vi "Handle Last Ack Core.vi"(4 "error in (no error)":errorcluster, 6 "Last Ack":refnum<class "Last Ack.lvclass">, 7 "Caller in":refnum<class "Caller.lvclass">) -> (0 "error out":errorcluster, 3 "Caller out":refnum<class "Caller.lvclass">)   [LabVIEW 2020, in "Caller.lvlib" / "Caller.lvclass"]
doc: "(<B>Filename</B>: Actor Framework.lvlib:Actor.lvclass:Handle Last Ack Core.vi)\n\nDefines how the caller actor responds to the Last Ack message from a nested actor. The Last Ack message is the final message a nested actor sends to its caller before it shuts down. The message contains information about the final state of the nested actor.\n\nBy default, this method does nothing except return any error the nested actor sent. A descendant class may override this method to define behavior."
uses:
  Caller.lvclass
  <vilib>/ActorFramework/LastAck/Last Ack.lvclass
  Nested/Nested.lvclass
  <vilib>/ActorFramework/LastAck/Last Ack.lvclass/Last Ack.ctl
  Nested/Nested.lvclass/Nested.ctl
  Caller.lvclass/Caller.ctl
  <vilib>/ActorFramework/Message Enqueuer/Message Enqueuer.lvclass/Message Enqueuer.ctl
  399a52ab-de9c-4f47-9720-846dc4beb769.vi
  Nested/Read Numeric.vi
  399a52ab-de9c-4f47-9720-846dc4beb769.vi/d4db2432-cc9c-482c-8957-dac855435ef6.vi
  399a52ab-de9c-4f47-9720-846dc4beb769.vi/86fbf154-bd7b-49a2-8ab2-a837b2a95f24.vi
  399a52ab-de9c-4f47-9720-846dc4beb769.vi/3b95b01e-1ec2-4565-bcd9-7606a5281010.vi
  399a52ab-de9c-4f47-9720-846dc4beb769.vi/96a08935-737a-44b2-979c-a81d56408f7e.vi
  <vilib>/ActorFramework/Message Enqueuer/Enqueue.vi
  399a52ab-de9c-4f47-9720-846dc4beb769.vi/d4db2432-cc9c-482c-8957-dac855435ef6.vi/6eaecd13-6e48-4772-a921-b51ebdf84d88.vi
  399a52ab-de9c-4f47-9720-846dc4beb769.vi/d4db2432-cc9c-482c-8957-dac855435ef6.vi/d2d5f2b7-06f4-47f6-971c-049c3fdbb653.vi
  399a52ab-de9c-4f47-9720-846dc4beb769.vi/3b95b01e-1ec2-4565-bcd9-7606a5281010.vi/6eaecd13-6e48-4772-a921-b51ebdf84d88.vi
  399a52ab-de9c-4f47-9720-846dc4beb769.vi/3b95b01e-1ec2-4565-bcd9-7606a5281010.vi/d2d5f2b7-06f4-47f6-971c-049c3fdbb653.vi
  399a52ab-de9c-4f47-9720-846dc4beb769.vi/96a08935-737a-44b2-979c-a81d56408f7e.vi/6eaecd13-6e48-4772-a921-b51ebdf84d88.vi
  399a52ab-de9c-4f47-9720-846dc4beb769.vi/96a08935-737a-44b2-979c-a81d56408f7e.vi/d2d5f2b7-06f4-47f6-971c-049c3fdbb653.vi
  Caller Messages/UpdateCPTNested Msg/UpdateCPTNested Msg.lvclass
  C:/Program Files/National Instruments/LabVIEW 2020/vi.lib/ActorFramework/Message/Message.lvclass
  <vilib>/ActorFramework/Message Priority Queue/Priority Enqueue.vi
  <vilib>/ActorFramework/Actor/Actor.lvclass
  <vilib>/Comparison/Less/Less Functor/Less Functor.lvclass
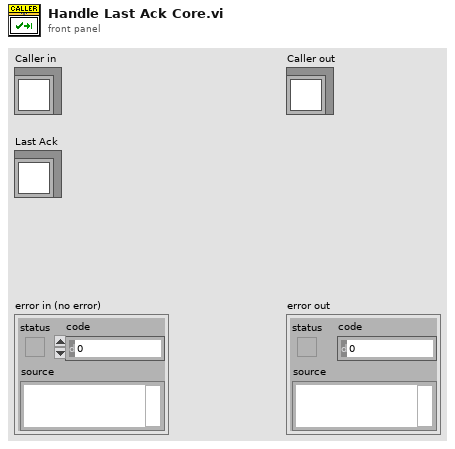
[diagram p1: front panel]
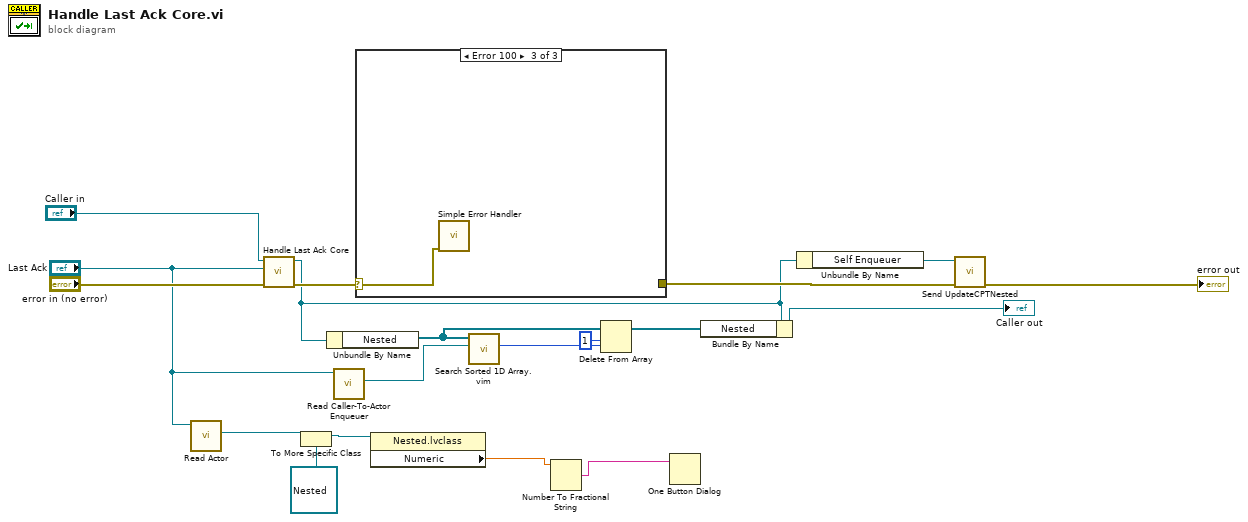
[diagram p0: block diagram]
diagram:
  n1 = call <vilib>:"Read Actor.vi"("Last Ack"="Last Ack") -> ("Actor"=w3:refnum<class "Actor.lvclass">)  [unwired: 10 in]
  n2 = call-parent "Handle Last Ack Core.vi"("error in (no error)"="error in (no error)", "Last Ack"="Last Ack", "Actor in"="Caller in") -> ("error out"=w9:errorcluster, "Actor out"=w7:refnum<class "Caller.lvclass">)  [unwired: 3 in]
  n3 = To More Specific Class(target class=refnum<class "Nested.lvclass"> refnum ("Nested.lvlib:Nested.lvclass"), reference=w3) -> (specific class reference=w4:refnum<class "Nested.lvclass">)  [unwired: 1 in, 1 out]
  n4 = Unbundle By Name(w7) -> ("Nested"=w14:refnum<class "Message Enqueuer.lvclass">[])
  n5 = call <vilib>:"Read Caller-To-Actor Enqueuer.vi"("Last Ack"="Last Ack") -> ("Caller-to-Actor Enqueuer"=w15:refnum<class "Message Enqueuer.lvclass">)  [unwired: 10 in]
  n6 = case shown="Error 100" w9 {
    selector: w9 -> [w20 w21 w22]
    tunnel: [w20 w21 _] -> w8
    frame No Error {
    }
    frame Default {
    }
    frame Error {
      n7 = call <vilib>:"Simple Error Handler.vi"("error in (no error)"=w22) -> ()  [unwired: 4 in, 5 out]
    }
  }
  n8 = property class="Nested.lvclass"(reference=w4) -> ("Numeric"=w2:dbl)  [unwired: 1 in, 2 out]
  n9 = call "Search Sorted 1D Array.vim"("element"=w15, "sorted 1D array"=w14) -> ("nearest index"=w13:i32)  [unwired: 8 in, 1 out]
  n10 = Number To Fractional String(number=w2) -> (F-format string=w1:string)  [unwired: 3 in]
  n11 = Delete From Array(array=w14, length=1, index=w13) -> (array with subset deleted=w10:refnum<class "Message Enqueuer.lvclass">[])  [unwired: 1 out]
  n12 = One Button Dialog(message=w1) -> ()  [unwired: 1 in, 1 out]
  n13 = Bundle By Name(cluster=w7, "Nested"=w10) -> (→"Caller out":refnum<class "Caller.lvclass">)
  n14 = Unbundle By Name(w7) -> ("Self Enqueuer"=w16:refnum<class "Message Enqueuer.lvclass">)
  n15 = call "Send UpdateCPTNested.vi"("error in (no error)"=w8, "Message Enqueuer"=w16) -> ("error out"=→"error out":errorcluster)  [unwired: 8 in, 1 out]
